vi "Array-Parse from string.vi"(7 "String":string, 11 "error in (no error)":errorcluster) -> (8 "Array":dbl[](array[numeric]), 15 "error out":errorcluster)   [LabVIEW 2020]
uses:
  <vilib>/regexp/Match Regular Expression.xnode
  <vilib>/gmath/NI_Gmath.lvlib
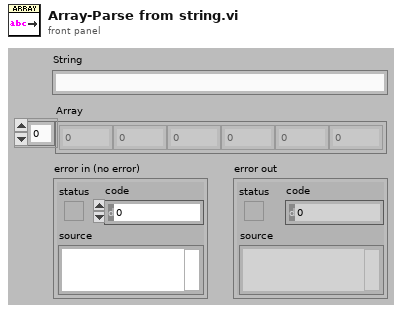
[diagram p1: front panel]
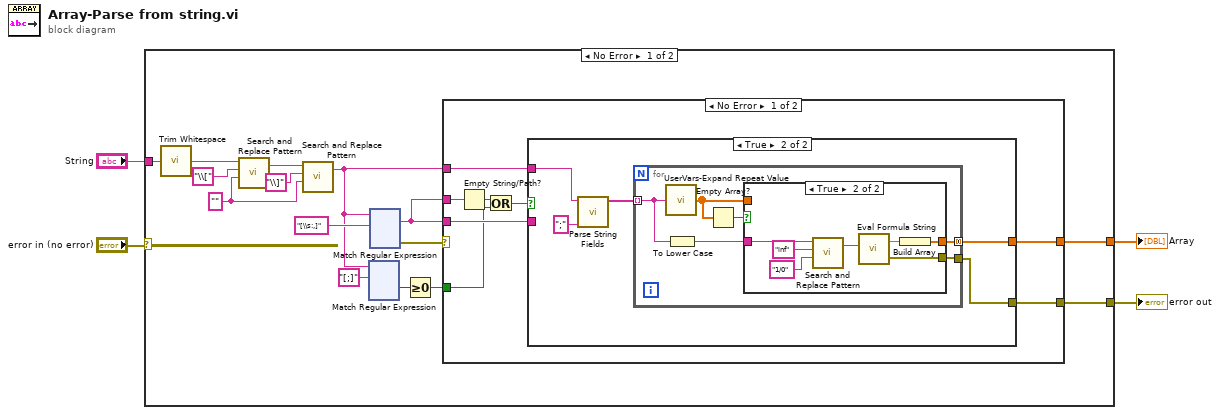
[diagram p0: block diagram]
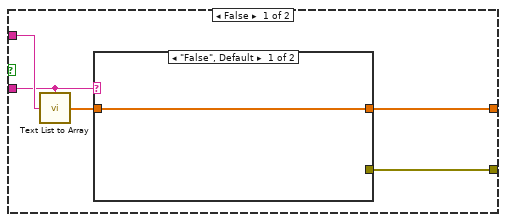
[diagram p2: hidden frame]
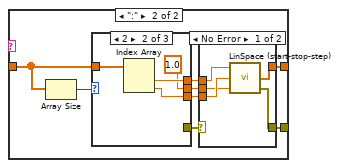
[diagram p3: hidden frame]
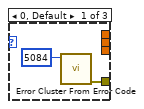
[diagram p5: hidden frame]
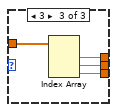
[diagram p6: hidden frame]
diagram:
  n1 = case shown="No Error" "error in (no error)" {
    selector: "error in (no error)" -> [_ w300]
    tunnel: [w15 w300] -> w3
    tunnel: "String" -> [w6 _]
    tunnel: [w16 _] -> w1
    frame No Error {
      w12 = "" ("replace string (\"\")")
      n2 = call <vilib>:"Trim Whitespace.vi"("string"=w6) -> ("trimmed string"=w5:string)  [unwired: 1 in]
      n3 = call <vilib>:"Search and Replace Pattern.vi"("string"=w5, "regular expression (\"\")"="\\[" ("regular expression (\"\")"), "replace string (\"\")"=w12) -> ("result string"=w11:string)  [unwired: 2 in, 1 out]
      n4 = call <vilib>:"Search and Replace Pattern.vi"("string"=w11, "regular expression (\"\")"="\\]" ("regular expression (\"\")"), "replace string (\"\")"=w12) -> ("result string"=w10:string)  [unwired: 2 in, 1 out]
      n5 = xnode "Match Regular Expression"("input string"=w10, "regular expression"="[;]") -> ("offset past match"=w8:i32)  [unwired: 4 in, 4 out]
      n6 = xnode "Match Regular Expression"("input string"=w10, "regular expression"="[\\s:,]") -> ("whole match"=w17:string, "error out"=w18:errorcluster)  [unwired: 4 in, 3 out]
      n7 = Greater Or Equal To 0?(x=w8) -> (x >= 0?=w7:bool)
      n8 = case shown="No Error" w18 {
        selector: w18 -> [_ w188]
        tunnel: w17 -> [w138 _]
        tunnel: w17 -> [w136 _]
        tunnel: w10 -> [w135 _]
        tunnel: [w134 _] -> w16
        tunnel: [w133 w188] -> w15
        tunnel: w7 -> [w131 _]
        frame No Error {
          n9 = Empty String/Path?(string/path=w138) -> (empty?=w137:bool)
          n10 = Or(x=w137, y=w131) -> (x .or. y?=w132:bool)
          n11 = case shown="True" w132 {
            tunnel: w136 -> [w141 _]
            tunnel: w135 -> [w143 w172]
            tunnel: [w140 w170] -> w134
            tunnel: [w139 w173] -> w133
            frame False {
              n12 = call "Text List to Array.vi"("delimiter (;)"=w141, "text list"=w143) -> ("array"=w142:dbl[])  [unwired: 2 in]
              n13 = case shown="\"False\", Default" w141 {
                tunnel: w142 -> [w144 w147]
                tunnel: [w144 w149] -> w140
                tunnel: [_ w146] -> w139
                frame "False", Default {
                }
                frame ":" {
                  n14 = Array Size(array=w147) -> (size(s)=w148:i32)
                  n15 = case shown="2" w148 {
                    tunnel: w147 -> [_ w164 w168]
                    tunnel: [_ w163 w167] -> w152
                    tunnel: [_ w162 w166] -> w151
                    tunnel: [_ 1.0 w165] -> w150
                    tunnel: [w160 _ _] -> w145
                    frame 0, Default {
                      n16 = call <vilib>:"Error Cluster From Error Code.vi"("error code (0)"=5084) -> ("error out"=w160:errorcluster)  [unwired: 8 in]
                    }
                    frame 2 {
                      n17 = Index Array(array=w164) -> (element #1=w163:dbl, element #2=w162:dbl)  [unwired: 2 in]
                    }
                    frame 3 {
                      n18 = Index Array(array=w168) -> (element #1=w167:dbl, element #2=w165:dbl, element #3=w166:dbl)  [unwired: 3 in]
                    }
                  }
                  n19 = case shown="No Error" w145 {
                    selector: w145 -> [_ w158]
                    tunnel: w152 -> [w157 _]
                    tunnel: w151 -> [w156 _]
                    tunnel: w150 -> [w155 _]
                    tunnel: [w154 _] -> w149
                    tunnel: [w153 w158] -> w146
                    frame No Error {
                      n20 = call "LinSpace (start-stop-step).vi"("Step"=w155, "Stop"=w156, "Start"=w157) -> ("error out"=w153:errorcluster, "Array"=w154:dbl[])  [unwired: 1 in]
                    }
                    frame Error {
                    }
                  }
                }
              }
            }
            frame True {
              n21 = call "Parse String Fields.vi"("Separator"=";", "String"=w172) -> ("Fields"=w169:string[])  [unwired: 8 in, 1 out]
              n22 = for {
                tunnel: [w179] -> w170 mode=concatenating
                tunnel: [w178] -> w173
                tunnel: w169 -> [w175] mode=indexing
                n23 = call "UserVars-Expand Repeat Value.vi"("Expression"=w175) -> ("repeated values"=w177:dbl[])  [unwired: 14 in]
                n24 = To Lower Case(string=w175) -> (all lower case string=w174:string)
                n25 = Empty Array?(array=w177) -> (empty?=w176:bool)
                n26 = case shown="True" w176 {
                  tunnel: [w180 w185] -> w179
                  tunnel: [_ w186] -> w178
                  tunnel: w177 -> [w180 _]
                  tunnel: w174 -> [_ w184]
                  frame False {
                  }
                  frame True {
                    n27 = call <vilib>:"Search and Replace Pattern.vi"("string"=w184, "regular expression (\"\")"="inf" ("regular expression (\"\")"), "replace string (\"\")"="1/0" ("replace string (\"\")")) -> ("result string"=w183:string)  [unwired: 2 in, 1 out]
                    n28 = call <vilib>:"Eval Formula String.vi"("formula"=w183) -> ("error out"=w186:errorcluster, "y value"=w187:dbl)  [unwired: 1 in]
                    n29 = Build Array(w187) -> (w185:dbl[])
                  }
                }
              }
            }
          }
        }
        frame Error {
        }
      }
    }
    frame Error {
    }
  }
  "error out" <- w3
  "Array" <- w1
